vi "NI 9217_TASK_PT100.vi"(8 "error in":errorcluster, 11 "MODULE NAME":string) -> (0 "error out":errorcluster, 3 "task out":refnum<k21>)   [LabVIEW 2019]
uses:
  <vilib>/DAQmx/create/channels.llb/DAQmx Create Channel (AI-Temperature-RTD).vi
  <vilib>/DAQmx/configure/timing.llb/DAQmx Timing (Sample Clock).vi
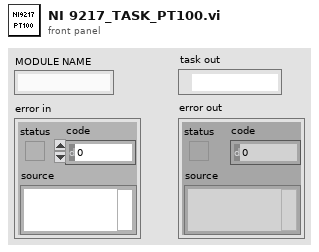
[diagram p1: front panel]
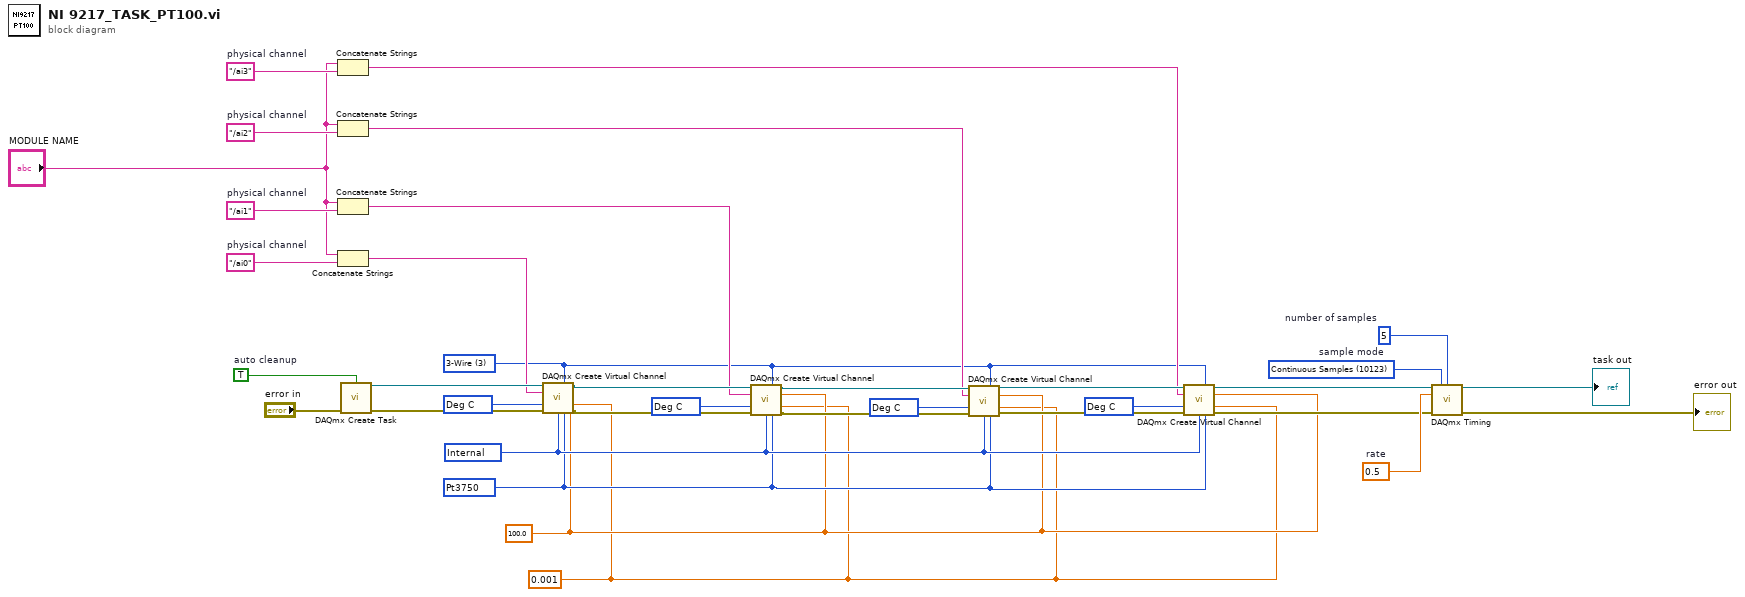
[diagram p0: block diagram]
diagram:
  w2 = 0.001 ("current excitation value")
  w3 = 100.0 ("r0")
  w11 = 10123 items=["Finite Samples"=10178, "Continuous Samples"=10123, "Hardware Timed Single Point"=12522]  # sample mode
  w12 = 5  # number of samples
  w13 = 0.5  # rate
  w19 = 10143 items=["Deg C"=10143, "Deg F"=10144, "Kelvins"=10325, "Deg R"=10145, "From Custom Scale"=10065] ("units")
  w22 = 10143 items=["Deg C"=10143, "Deg F"=10144, "Kelvins"=10325, "Deg R"=10145, "From Custom Scale"=10065] ("units")
  w25 = 10143 items=["Deg C"=10143, "Deg F"=10144, "Kelvins"=10325, "Deg R"=10145, "From Custom Scale"=10065] ("units")
  w31 = "/ai3"  # physical channel
  w30 = "/ai2"  # physical channel
  w29 = "/ai1"  # physical channel
  w28 = "/ai0"  # physical channel
  w34 = TRUE  # auto cleanup
  w6 = 3 items=["2-Wire"=2, "3-Wire"=3, "4-Wire"=4] ("resistance configuration")
  w35 = 10143 items=["Deg C"=10143, "Deg F"=10144, "Kelvins"=10325, "Deg R"=10145, "From Custom Scale"=10065] ("units")
  w5 = 10200 items=["Internal"=10200, "External"=10167, "None"=10230] ("current excitation source")
  w4 = 12481 items=["Pt3750"=12481, "Pt3851"=10071, "Pt3911"=12482, "Pt3916"=10069, "Pt3920"=10053, "Pt3928"=12483, "Custom"=10137] ("rtd type")
  n1 = Concatenate Strings("MODULE NAME", w31) -> (w14:string)
  n2 = Concatenate Strings("MODULE NAME", w30) -> (w15:string)
  n3 = Concatenate Strings("MODULE NAME", w29) -> (w16:string)
  n4 = Concatenate Strings("MODULE NAME", w28) -> (w26:string)
  n5 = call <vilib>:"DAQmx Create Task.vi"("auto cleanup"=w34, "error in"="error in") -> ("task out"=w32:refnum<k21>, "error out"=w33:errorcluster)  [unwired: 12 in]
  n6 = call-poly <vilib>:"DAQmx Create Virtual Channel.vi"("task in"=w32, "resistance configuration"=w6, "physical channels"=w26, "r0"=w3, "units"=w35, "current excitation value"=w2, "error in"=w33, "current excitation source"=w5, "rtd type"=w4) -> ("task out"=w24:refnum<k21>, "error out"=w23:errorcluster)  [unwired: 5 in]
  n7 = call-poly <vilib>:"DAQmx Create Virtual Channel.vi"("task in"=w24, "resistance configuration"=w6, "physical channels"=w16, "r0"=w3, "units"=w25, "current excitation value"=w2, "error in"=w23, "current excitation source"=w5, "rtd type"=w4) -> ("task out"=w21:refnum<k21>, "error out"=w20:errorcluster)  [unwired: 5 in]
  n8 = call-poly <vilib>:"DAQmx Create Virtual Channel.vi"("task in"=w21, "resistance configuration"=w6, "physical channels"=w15, "r0"=w3, "units"=w22, "current excitation value"=w2, "error in"=w20, "current excitation source"=w5, "rtd type"=w4) -> ("task out"=w18:refnum<k21>, "error out"=w17:errorcluster)  [unwired: 5 in]
  n9 = call-poly <vilib>:"DAQmx Create Virtual Channel.vi"("task in"=w18, "resistance configuration"=w6, "physical channels"=w14, "r0"=w3, "units"=w19, "current excitation value"=w2, "error in"=w17, "current excitation source"=w5, "rtd type"=w4) -> ("task out"=w9:refnum<k21>, "error out"=w10:errorcluster)  [unwired: 5 in]
  n10 = call-poly <vilib>:"DAQmx Timing.vi"("task/channels in"=w9, "sample mode"=w11, "samples per channel"=w12, "rate"=w13, "error in"=w10) -> ("task out"=→"task out":refnum<k21>, "error out"=→"error out":errorcluster)  [unwired: 9 in]
